vi "ADO Connection Insert Data.vi"(4 "use file? (F)":bool, 5 "create table? (F)":bool, 6 "flatten cluster? (F)":bool, 7 "table":string, 8 "error in (no error)":errorcluster caption="错误输入（无错误）", 9 "data":variant, 10 "columns":string[](array[string]), 11 "Database Connection 输入":refnum<class "Database Connection.lvclass"> caption="DNL_LabVIEW Object in") -> (0 "error out":errorcluster caption="错误输出", 2 "Database Command 输出":refnum<class "Database Command.lvclass">, 3 "Database Connection 输出":refnum<class "Database Connection.lvclass"> caption="DNL_LabVIEW Object out")   [LabVIEW 2011, in "Database Connection.lvclass"]
uses:
  Database Connection.lvclass
  Command/Database Command.lvclass
  <vilib>/addons/database/Auxilliary.llb/DB Tools Parameter Info.ctl
  <vilib>/addons/database/Auxilliary.llb/DB Tools DataTypes.ctl
  <vilib>/addons/database/Auxilliary.llb/DB Tools Parameter Dir.ctl
  <vilib>/addons/database/NI_Database_API.lvlib
panel:
  out "parameters out":T1[](array[typedef])
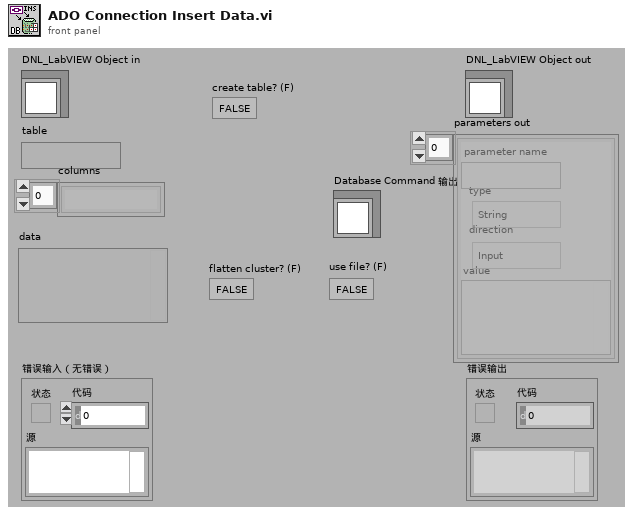
[diagram p1: front panel]
types:
  T1 = typedef "NI_Database_API.lvlib/DB Tools Parameter Info.ctl" = cluster{"parameter name":string, "type":T2, "direction":T3, "value":variant}
  T2 = typedef "NI_Database_API.lvlib/DB Tools DataTypes.ctl" = enum16{"String", "Long (I32)", "Single (SGL)", "Double (DBL)", "Date/Time", "Binary"}
  T3 = typedef "NI_Database_API.lvlib/DB Tools Parameter Dir.ctl" = enum32{"Input", "Output", "Input/Output", "Return Value"}
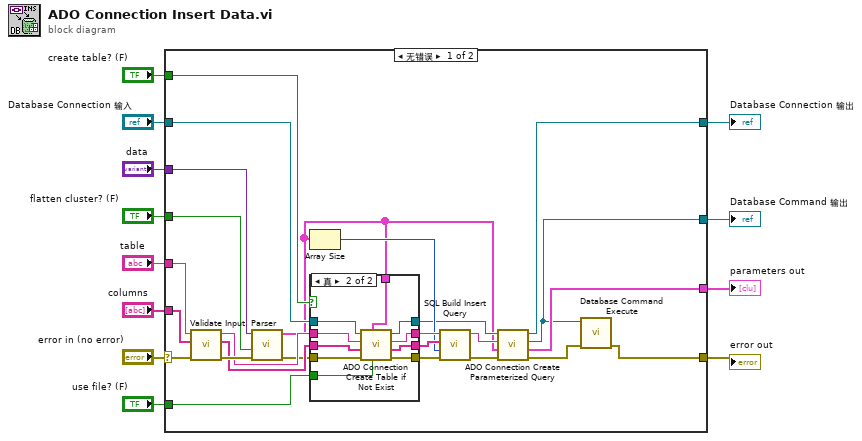
[diagram p0: block diagram]
diagram:
  n1 = case shown="无错误" "error in (no error)" {
    selector: "error in (no error)" -> [w35 w53]
    tunnel: [w14 w53] -> w11
    tunnel: [w20 w52] -> w9
    tunnel: "Database Connection 输入" -> [w28 w52]
    tunnel: "table" -> [w37 _]
    tunnel: "columns" -> [w36 _]
    tunnel: "data" -> [w34 _]
    tunnel: "flatten cluster? (F)" -> [w33 _]
    tunnel: "create table? (F)" -> [w18 _]
    tunnel: [w16 _] -> w3
    tunnel: [w19 _] -> w2
    tunnel: "use file? (F)" -> [w17 _]
    frame No Error {
      n2 = call "Validate Input.vi"("error in (no error)"=w35, "columns"=w36, "table"=w37) -> ("error out"=w32:errorcluster, "columns out"=w30:string[], "table out"=w31:string)  [unwired: 6 in]
      n3 = call "Parser.vi"("error in (no error)"=w32, "flatten cluster? (F)"=w33, "variant"=w34) -> ("error out"=w29:errorcluster, "parameters"=w13:T1[])  [unwired: 7 in]
      n4 = Array Size(array=w13) -> (size(s)=w24:i32)
      n5 = case shown="真" w18 {
        tunnel: w31 -> [w41 w50]
        tunnel: w30 -> [w40 w49]
        tunnel: w29 -> [w38 w51]
        tunnel: w28 -> [w39 w48]
        tunnel: [w39 w47] -> w23
        tunnel: [w41 w46] -> w27
        tunnel: [w40 w45] -> w26
        tunnel: [w38 w44] -> w25
        tunnel: w17 -> [_ w43]
        tunnel: w13 -> [_ w42]
        frame False {
        }
        frame True {
          n6 = call "ADO Connection Create Table if Not Exist.vi"("use file? (F)"=w43, "parameters"=w42, "error in (no error)"=w51, "columns"=w49, "table name"=w50, "Database Connection 输入"=w48) -> ("error out"=w44:errorcluster, "columns out"=w45:string[], "table"=w46:string, "Database Connection 输出"=w47:refnum<class "Database Connection.lvclass">)  [unwired: 2 in]
        }
      }
      n7 = call "SQL Build Insert Query.vi"("error in (no error)"=w25, "num parameters"=w24, "columns"=w26, "table name"=w27) -> ("error out"=w21:errorcluster, "insert query"=w22:string)  [unwired: 6 in]
      n8 = call "ADO Connection Create Parameterized Query.vi"("error in (no error)"=w21, "parameters"=w13, "SQL query"=w22, "Database Connection 输入"=w23) -> ("error out"=w15:errorcluster, "parameters out"=w19:T1[], "Database Command 输出"=w16:refnum<class "Database Command.lvclass">, "Database Connection 输出"=w20:refnum<class "Database Connection.lvclass">)  [unwired: 4 in]
      n9 = call "Database Command Execute.vi"("error in (no error)"=w15, "Database Command 输入"=w16) -> ("error out"=w14:errorcluster)  [unwired: 7 in, 2 out]
    }
    frame Error {
    }
  }
  "error out" <- w11
  "Database Connection 输出" <- w9
  "Database Command 输出" <- w3
  "parameters out" <- w2
